vi "写文件main.vi"(9 "下载路径":path=path "D:/项目/MPZ2006固态源/数据模版/参数表格文件样例.xlsx", 11 "VISA资源名称":refnum<visa-resource-name>="COM3") -> (2 "消息":string, 3 "VISA资源名称 2":refnum<visa-resource-name>)   [LabVIEW 2015]
uses:
  Globle.vi
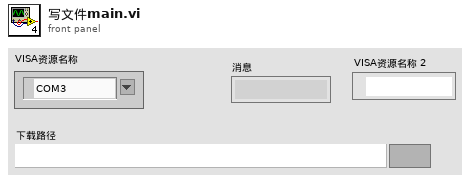
[diagram p1: front panel]
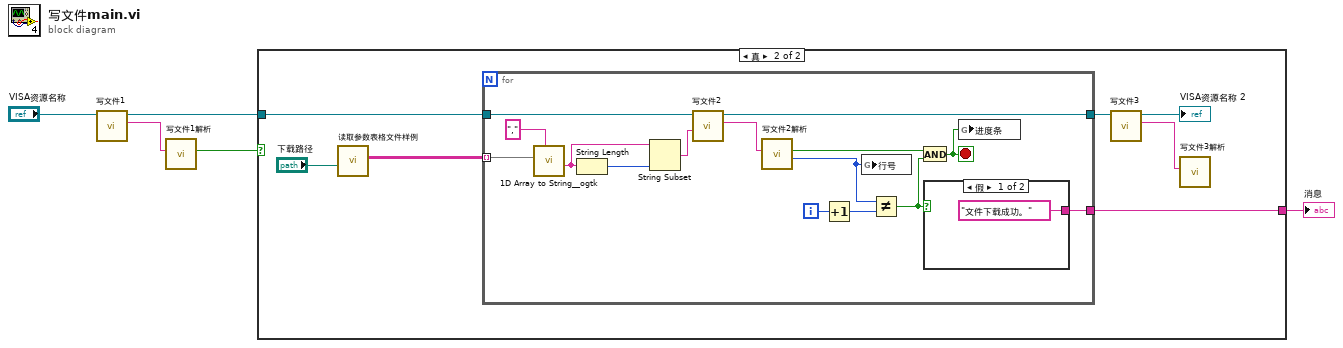
[diagram p0: block diagram]
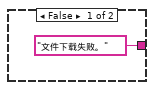
[diagram p2: hidden frame]
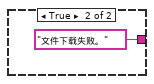
[diagram p3: hidden frame]
diagram:
  n1 = call "写文件1.vi"("VISA资源名称"="VISA资源名称") -> ("响应"=w4:string, "VISA资源名称 2"=w2:refnum<visa-resource-name>)  [unwired: 9 in]
  n2 = call "写文件1解析.vi"("响应"=w4) -> ("响应"=w5:bool)  [unwired: 10 in]
  n3 = case shown="真" w5 {
    tunnel: w2 -> [_ w11]
    tunnel: ["文件下载失败。" ("消息") w10] -> w1
    frame False {
    }
    frame True {
      n4 = call "读取参数表格文件样例.vi"("下载路径"="下载路径") -> ("data"=w12:string[][])  [unwired: 10 in]
      n5 = for {
        tunnel: w12 -> [w27] mode=indexing
        tunnel: w11 -> [w25]
        tunnel: [w22] -> w10
        tunnel: [w19] -> w8
        i -> [w24]
        stop <- w17 stop-if-true
        n6 = call <userlib>:"1D Array to String__ogtk.vi"("delimiter (Tab)"=",", "Array of Strings"=w27) -> ("delimited string"=w16:string)  [unwired: 9 in]
        n7 = String Length(string=w16) -> (length=w14:i32)
        n8 = String Subset(string=w16, length (rest)=w14) -> (substring=w15:string)  [unwired: 1 in]
        n9 = call "写文件2.vi"("参数"=w15, "VISA资源名称"=w25) -> ("响应"=w28:string, "VISA资源名称 2"=w19:refnum<visa-resource-name>)  [unwired: 8 in]
        n10 = call "写文件2解析.vi"("响应"=w28) -> ("返回行号"=w18:u32, "响应"=w21:bool)  [unwired: 9 in]
        n11 = Increment(x=w24) -> (x+1=w23:i32)
        n12 = global write "Globle.vi" "行号"(w18) -> ()
        n13 = Not Equal?(x=w18, y=w23) -> (x != y?=w20:bool)
        n14 = And(x=w21, y=w20) -> (x .and. y?=w17:bool)
        n15 = case shown="假" w20 {
          tunnel: ["文件下载成功。" ("消息") "文件下载失败。" ("消息")] -> w22
          frame False {
          }
          frame True {
          }
        }
        n16 = global write "Globle.vi" "进度条"(w17) -> ()
      }
      n17 = call "写文件3.vi"("VISA资源名称"=w8) -> ("响应"=w9:string, "VISA资源名称 2"=→"VISA资源名称 2":refnum<visa-resource-name>)  [unwired: 9 in]
      n18 = call "写文件3解析.vi"("响应"=w9) -> ()  [unwired: 10 in, 1 out]
    }
  }
  "消息" <- w1
